vi "WritebyRefNumArr.vi"(8 "error in":errorcluster caption="entrée d'erreur", 10 "Valeur":dbl, 11 "Ctrl Ref":refnum<vi>[](array[refnum])) -> (0 "error out":errorcluster caption="sortie d'erreur")   [LabVIEW 2010]
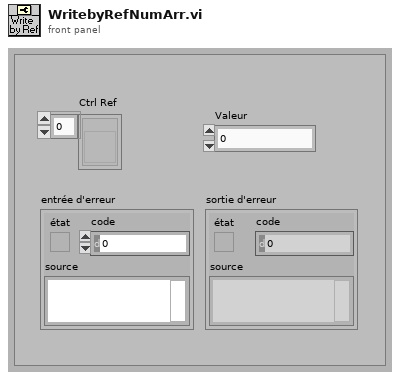
[diagram p1: front panel]
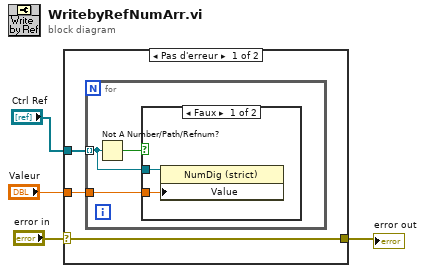
[diagram p0: block diagram]
diagram:
  n1 = case shown="Pas d'erreur" "error in" {
    selector: "error in" -> [w5 w13]
    tunnel: "Ctrl Ref" -> [w7 _]
    tunnel: "Valeur" -> [w6 _]
    tunnel: [w5 w13] -> w2
    frame No Error {
      n2 = for {
        tunnel: w7 -> [w9] mode=indexing
        tunnel: w6 -> [w8]
        n3 = Not A Number/Path/Refnum?(number/path/refnum=w9) -> (NaN/Path/Refnum?=w10:bool)
        n4 = case shown="Faux" w10 {
          tunnel: w9 -> [w12 _]
          tunnel: w8 -> [w11 _]
          frame False {
            n5 = property class="NumDig (strict)"(reference=w12, "Value"=w11) -> ()  [unwired: 1 in, 2 out]
          }
          frame True {
          }
        }
      }
    }
    frame Error {
    }
  }
  "error out" <- w2
